vi "Host - Configure Default Data.vi"(9 "DO":T1[](array[typedef]), 10 "DI":T1[](array[typedef]), 11 "Source":string[](array[string])) -> (2 "DO Data":cluster{"Names":string[], "Data":bool[]}[](array[cluster]), 3 "DI Data":cluster{bool[]}[](array[cluster]))   [LabVIEW 2021]
uses:
  Digital Output/Controls/DIO Configuration cluster.ctl
  Digital Output/Controls/DIO Interface Data.ctl
  Digital Output/SubVIs/Digital Dynamic Cluster.ctl
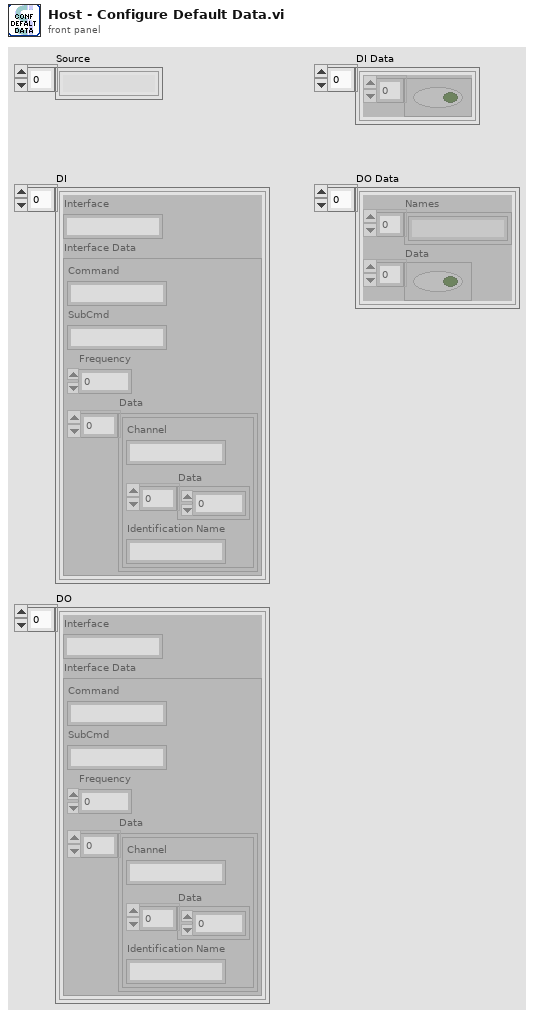
[diagram p1: front panel]
types:
  T1 = typedef "DIO Configuration cluster.ctl" = cluster{"Interface":string, "Interface Data":T2}
  T2 = typedef "DIO Interface Data.ctl" = cluster{"Command":string, "SubCmd":string, "Frequency":u16, "Data":T3[]}
  T3 = typedef "Digital Dynamic Cluster.ctl" = cluster{"Channel":string, "Data":u8[], "Identification Name":string}
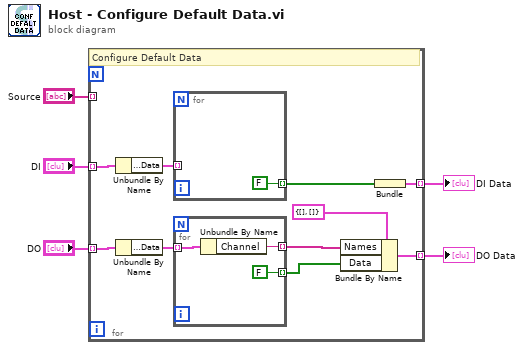
[diagram p0: block diagram]
diagram:
  n1 = for {
    tunnel: "DO" -> [w15] mode=indexing
    tunnel: [w10] -> w2 mode=indexing
    tunnel: "Source" -> [_] mode=indexing
    tunnel: "DI" -> [w9] mode=indexing
    tunnel: [w6] -> w4 mode=indexing
    # "Configure Default Data"
    n2 = Unbundle By Name(w9) -> ("Interface Data.Data"=w8:T3[])
    n3 = Unbundle By Name(w15) -> ("Interface Data.Data"=w14:T3[])
    n4 = for {
      tunnel: w8 -> [_] mode=indexing
      tunnel: [FALSE] -> w7 mode=indexing
    }
    n5 = for {
      tunnel: w14 -> [w19] mode=indexing
      tunnel: [FALSE] -> w12 mode=indexing
      tunnel: [w17] -> w11 mode=indexing
      n6 = Unbundle By Name(w19) -> ("Channel"=w17:string)
    }
    n7 = Bundle By Name(cluster=cluster{"Names":string[], "Data":bool[]} {"Names"=[], "Data"=[]}, "Names"=w11, "Data"=w12) -> (w10:cluster{"Names":string[], "Data":bool[]})
    n8 = Bundle(w7) -> (w6:cluster{bool[]})  [unwired: 1 in]
  }
  "DI Data" <- w4
  "DO Data" <- w2
